vi "Extract-elements-from-file.vi"(8 "error in (no error)":errorcluster, 11 "Reference in":T1) -> (0 "error out":errorcluster, 1 "Succes?":bool, 3 "Reference out":T1)   [LabVIEW 2013, in "MaterialCharacterization.lvlib" / "MC-ScanParser.lvclass"]
uses:
  MC-ScanParser.lvclass
  Object-reference.ctl
  SM1000-XML/Element-XML/Element-XML.lvclass
  SM1000-XML/Element-XML/XML-parser-state.ctl
  MC-ScanParser.lvclass/MC-ScanParser.ctl
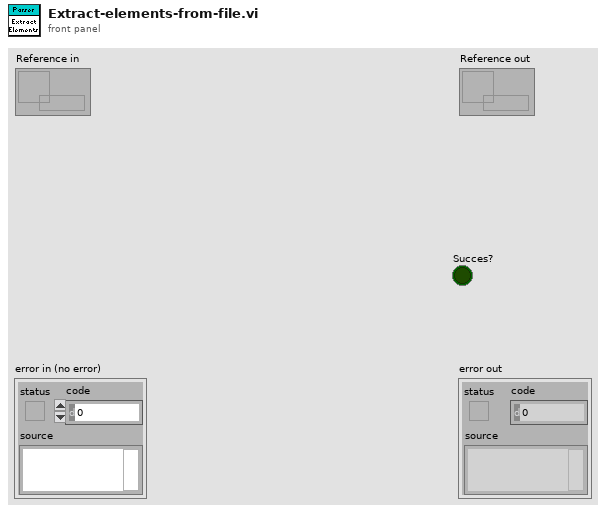
[diagram p1: front panel]
types:
  T1 = typedef "MaterialCharacterization.lvlib/MC-ScanParser.lvclass/Object-reference.ctl" = refnum<data-value>
  T2 = typedef "MaterialCharacterization.lvlib/Element-XML.lvclass/XML-parser-state.ctl" = cluster{"Current ItemID":u32, "Last parent ItemID":u32, "Current nesting level":i16, "Pending elements":refnum<class "Element-XML.lvclass">[]}
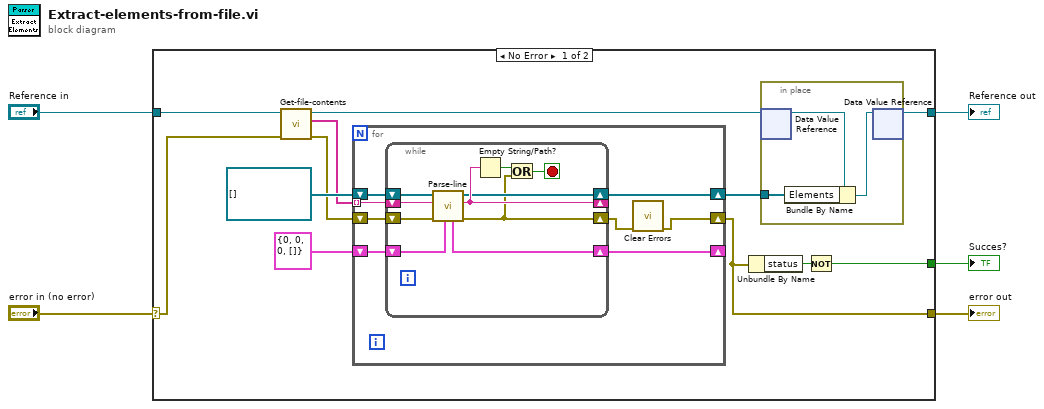
[diagram p0: block diagram]
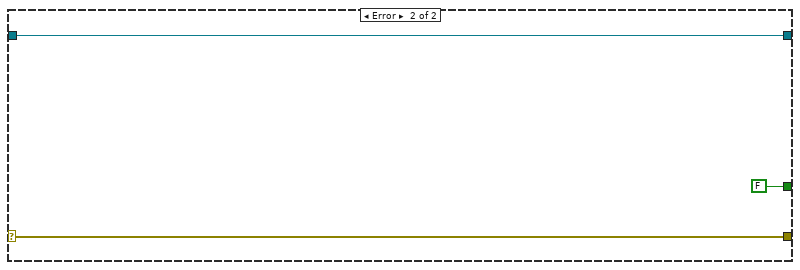
[diagram p2: hidden frame]
diagram:
  n1 = case shown="No Error" "error in (no error)" {
    selector: "error in (no error)" -> [w8 w40]
    tunnel: [w14 w40] -> w4
    tunnel: [w11 w41] -> w2
    tunnel: "Reference in" -> [w13 w41]
    tunnel: [w10 FALSE] -> w1
    frame No Error {
      n2 = call "Get-file-contents.vi"("error in (no error)"=w8, "Reference in"=w13) -> ("error out"=w7:errorcluster, "File contents"=w6:string[], "Reference out"=w9:T1)  [unwired: 7 in]
      n3 = for {
        tunnel: w6 -> [w28] mode=indexing
        shift-right: [w25] -> w12
        shift-left: refnum<class "Element-XML.lvclass">[] [] ("Elements in") -> [w27]
        shift-right: [w24] -> _
        shift-left: T2 {"Current ItemID"=0, "Last parent ItemID"=0, "Current nesting level"=0, "Pending elements"=[]} ("State data in") -> [w26]
        shift-right: [w21] -> w14
        shift-left: w7 -> [w23]
        n4 = while {
          shift-right: [w37] -> _
          shift-left: w28 -> [w38]
          shift-right: [w33] -> w24
          shift-left: w26 -> [w34]
          shift-right: [w35] -> w25
          shift-left: w27 -> [w36]
          shift-right: [w30] -> w22
          shift-left: w23 -> [w32]
          stop <- w29 stop-if-true
          n5 = call "Parse-line.vi"("State data in"=w34, "error in"=w32, "Line in"=w38, "Elements in"=w36) -> ("error IO"=w30:errorcluster, "Remaining line"=w37:string, "Elements"=w35:refnum<class "Element-XML.lvclass">[], "State data"=w33:T2)  [unwired: 4 in]
          n6 = Empty String/Path?(string/path=w37) -> (empty?=w31:bool)
          n7 = Or(x=w31, y=w30) -> (x .or. y?=w29:bool)
        }
        n8 = call <vilib>:"Clear Errors.vi"("error in (no error)"=w22) -> ("error out"=w21:errorcluster)  [unwired: 6 in]
      }
      n9 = Unbundle By Name(w14) -> ("status"=w15:bool)
      n10 = in-place {
        in-place-border: w12 -> [w19]
        n11 = in-place-dvr #1(w9) -> (w20:refnum<class "MC-ScanParser.lvclass">)  [unwired: 1 out]
        n12 = Bundle By Name(cluster=w20, "Elements"=w19) -> (w18:refnum<class "MC-ScanParser.lvclass">)
        n13 = in-place-dvr #1(w18) -> (w11:T1)  [unwired: 1 out]
      }
      n14 = Not(x=w15) -> (.not. x?=w10:bool)
    }
    frame Error {
    }
  }
  "error out" <- w4
  "Reference out" <- w2
  "Succes?" <- w1
